vi "Actor Core.vi"(8 "error in (no error)":errorcluster, 11 "Request in":refnum<class "RequestRestUI.lvclass">) -> (0 "error out":errorcluster, 3 "Actor out":refnum<class "Actor.lvclass">)   [LabVIEW 2015, in "RequestRestUI.lvclass"]
doc: "(<B>Filename</B>: Actor Framework.lvlib:Actor.lvclass:Actor Core.vi)\n\nReceives messages to the actor, reacts to them, and initiates any error handling that may shut the actor down.\n\nDescendant classes may override this VI to append parallel tasks for the actor to complete while it handles messages. Overrides use the Call Parent Method node."
uses:
  RequestRestUI.lvclass
  <vilib>/ActorFramework/Stop Msg/Stop Msg.lvclass
  <vilib>/ActorFramework/Actor/Actor.lvclass
  Messages/Add Member to Database_Msg/Add Member to Database_Msg.lvclass
  PluginWithDatabase/PluginWithDatabase.lvclass
  typedef/RequestRestInfo.ctl
panel:
  in  "Request":bool
  in  "RequestRestInfo":T1
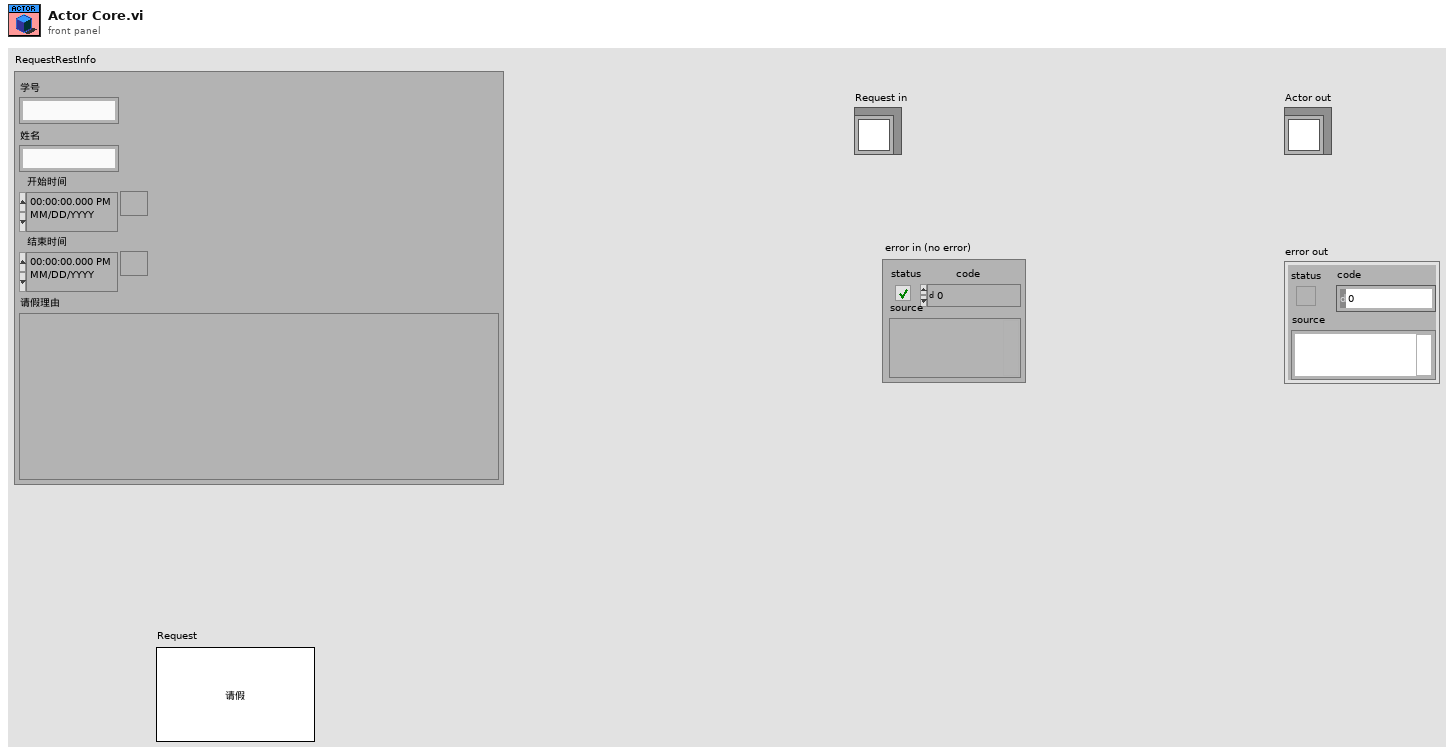
[diagram p1: front panel]
types:
  T1 = typedef "RequestRestUI.lvclass/RequestRestInfo.ctl" = cluster{"学号":string, "姓名":string, "开始时间":timestamp, "结束时间":timestamp, "请假理由":string}
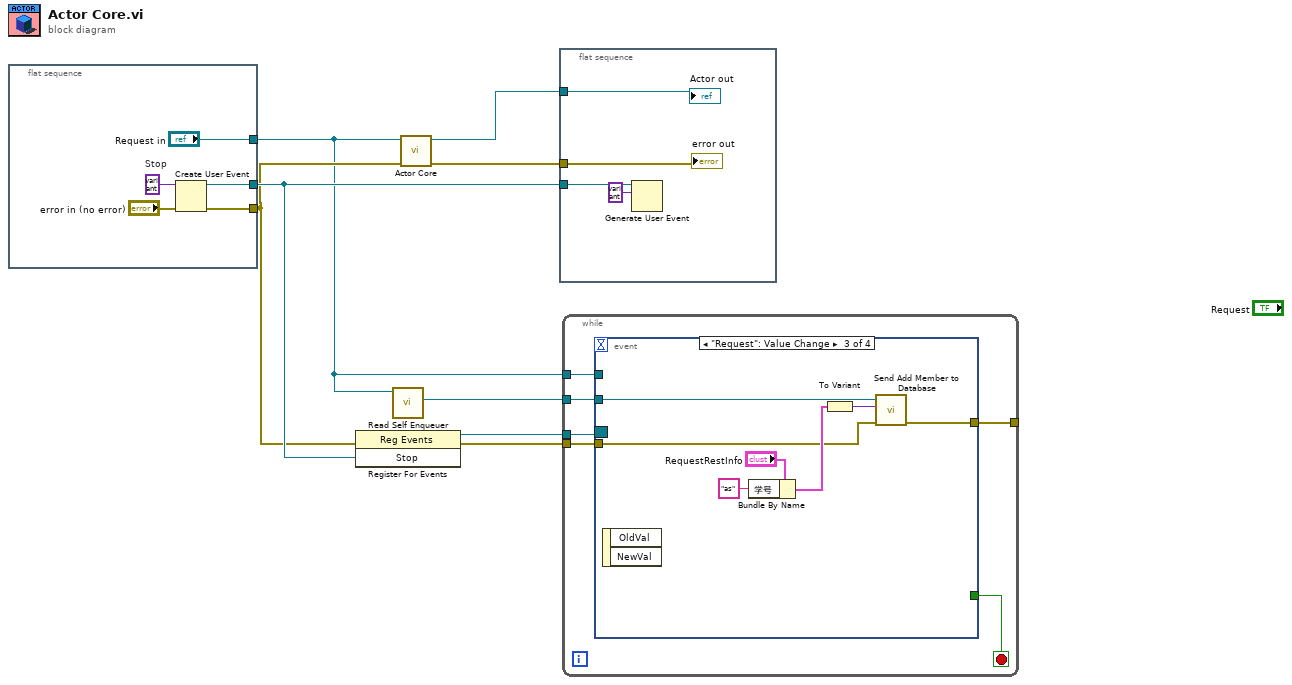
[diagram p0: block diagram]
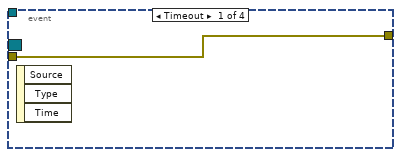
[diagram p2: hidden frame]
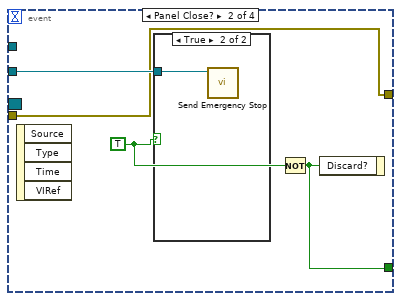
[diagram p3: hidden frame]
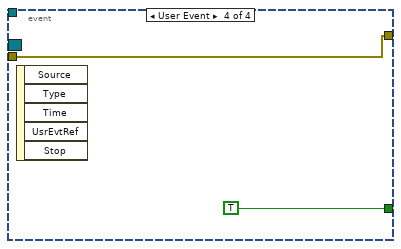
[diagram p5: hidden frame]
diagram:
  n1 = flat-sequence {
    tunnel: [w12] -> w5
    tunnel: [w11] -> w4
    tunnel: ["Request in"] -> w3
    frame #0 {
      w13 = variant  # Stop
      n2 = Create User Event(user event datatype=w13, error in="error in (no error)") -> (user event=w12:refnum<user-event>, error out=w11:errorcluster)
    }
  }
  n3 = register-events(error in=w4, w5) -> (reference out=w6:refnum<event-registration>, error out=w7:errorcluster)  [unwired: 1 in]
  n4 = call <vilib>:"Read Self Enqueuer.vi"("Actor"=w3) -> ("Self Enqueuer"=w8:refnum<class "Message Enqueuer.lvclass">)  [unwired: 10 in]
  n5 = call-parent "Actor Core.vi"("error in"=w4, "Actor in"=w3) -> ("error out"=w1:errorcluster, "Actor out"=w2:refnum<class "Actor.lvclass">)  [unwired: 8 in]
  n6 = flat-sequence {
    tunnel: w5 -> [w17]
    tunnel: w2 -> [w15]
    tunnel: w1 -> [w14]
    frame #0 {
      n7 = Generate User Event(user event=w17, event data cluster=variant ("event data")) -> ()  [unwired: 2 in, 2 out]
      "error out" <- w14
      "Actor out" <- w15
    }
  }
  n8 = while {
    tunnel: w6 -> [w23]
    tunnel: w7 -> [w19]
    tunnel: w8 -> [w22]
    tunnel: w3 -> [w21]
    tunnel: [w18] -> _
    stop <- w20 stop-if-true
    n9 = event shown="[2] \"Request\": Value Change" {
      selector: w23 -> [_ _ _ _]
      dyn-events: _ -> [_ _ _ _]
      timeout: _ -> [_ _ _ _]
      tunnel: w22 -> [_ w28 w33 _]
      tunnel: w21 -> [_ _ _ _]
      tunnel: [_ w26 _ TRUE] -> w20
      tunnel: w19 -> [w24 w25 w31 w37]
      tunnel: [w24 w25 w30 w37] -> w18
      event Timeout {
        n10 = event-data() -> ()  [unwired: 1 in, 3 out]
      }
      event Panel Close? {
        w27 = TRUE
        n11 = event-data() -> ()  [unwired: 1 in, 4 out]
        n12 = case shown="True" w27 {
          tunnel: w28 -> [_ w29]
          frame False {
          }
          frame True {
            n13 = call <vilib>:"Send Emergency Stop.vi"("Message Enqueuer"=w29) -> ()  [unwired: 10 in, 1 out]
          }
        }
        n14 = Not(x=w27) -> (.not. x?=w26:bool)
        n15 = event-data("Discard?"=w26) -> ()  [unwired: 1 in, 1 out]
      }
      event "Request": Value Change {
        n16 = event-data() -> ()  [unwired: 1 in, 2 out]
        n17 = Bundle By Name(cluster="RequestRestInfo", "学号"="as") -> (w34:T1)
        n18 = To Variant(anything=w34) -> (Variant=w32:variant)
        n19 = call "Send Add Member to Database.vi"("error in (no error)"=w31, "UI data"=w32, "Message Enqueuer"=w33) -> ("error out"=w30:errorcluster)  [unwired: 7 in, 1 out]
      }
      event User Event {
        n20 = event-data() -> ()  [unwired: 1 in, 5 out]
      }
    }
  }
